vi "Find available neighbours.vi"(11 "Points In":set{cluster{i32, i32}}(c389)) -> (3 "Points Out":set{cluster{i32, i32}}(c389))   [LabVIEW 2021]
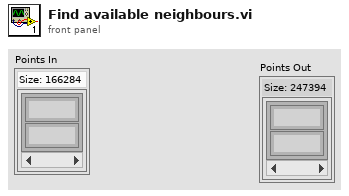
[diagram p1: front panel]
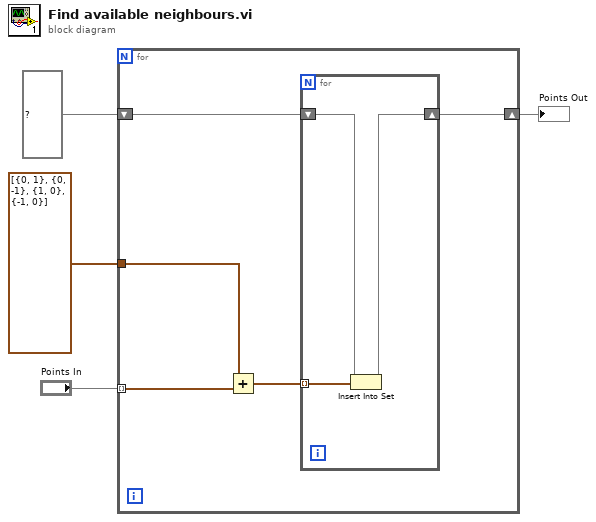
[diagram p0: block diagram]
diagram:
  n1 = for {
    tunnel: "Points In" -> [w8] mode=indexing
    tunnel: cluster{i32, i32}[] [{0, 1}, {0, -1}, {1, 0}, {-1, 0}] -> [w9]
    shift-right: [w5] -> w1
    shift-left: set{cluster{i32, i32}} {} ("set in") -> [w6]
    n2 = Add(x=w9, y=w8) -> (x+y=w7:cluster{i32, i32}[])
    n3 = for {
      tunnel: w7 -> [w12] mode=indexing
      shift-right: [w10] -> w5
      shift-left: w6 -> [w11]
      n4 = Insert Into Set(10:w12, 11:w11) -> (3:w10:set{cluster{i32, i32}})  [unwired: 1 out]
    }
  }
  "Points Out" <- w1
